vi "punto2.vi"() -> ()   [LabVIEW 2022 SP3]
uses:
  <vilib>/Instr/_visa.llb/VISA Configure Serial Port (Instr).vi
  <vilib>/addons/control/pid/pid.llb/PID (DBL).vi
  <vilib>/addons/control/pid/NI_PID_pid.lvlib
panel:
  in  "Potencia Manual":i16 min=0 max=100 step=1
  in  "Modo":bool=TRUE
  out "Input":cluster{i16}(graph)
  out "Velocidad":i32
  in  "PID gains":T1={"proportional gain (Kc)"=0.8, "integral time (Ti, min)"=0.053, "derivative time (Td, min)"=0.0} {"derivative time (Td, min)" format="%.3f"; "integral time (Ti, min)" format="%.3f"; "proportional gain (Kc)" format="%.3f"}
  in  "VISA resource name":refnum<visa-resource-name>
  in  "Stop Button":bool
  out "Output":cluster{i32, "Set Point":dbl}(graph)
  in  "Set Point":dbl
  # "INTEGRANTES"
  # "- SEBASTIÁN ALZATE SIERRA \n- GRACHI GONZALEZ PULGARIN \n- PABLO GARCÍA SUÁREZ"
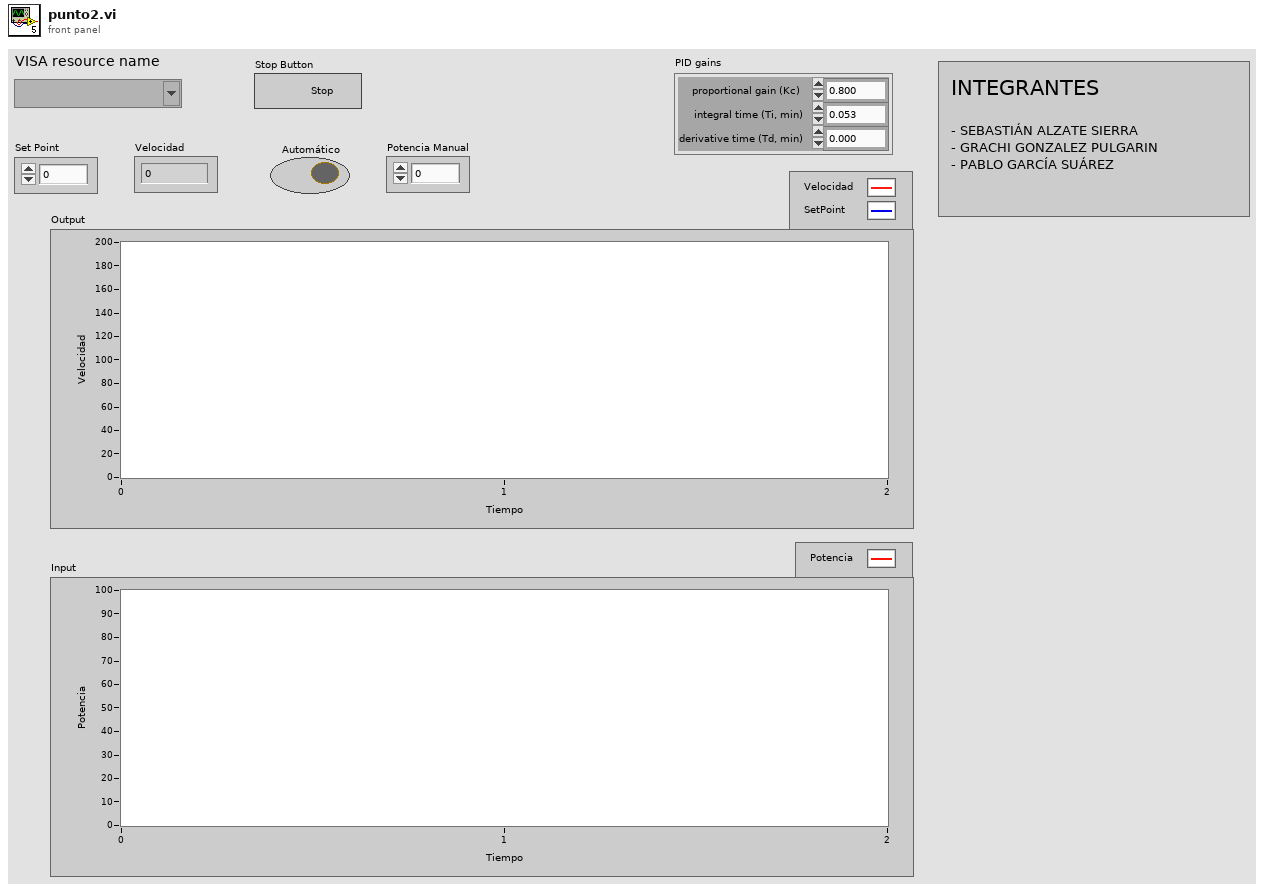
[diagram p1: front panel]
types:
  T1 = cluster{"proportional gain (Kc)":dbl, "integral time (Ti, min)":dbl, "derivative time (Td, min)":dbl}
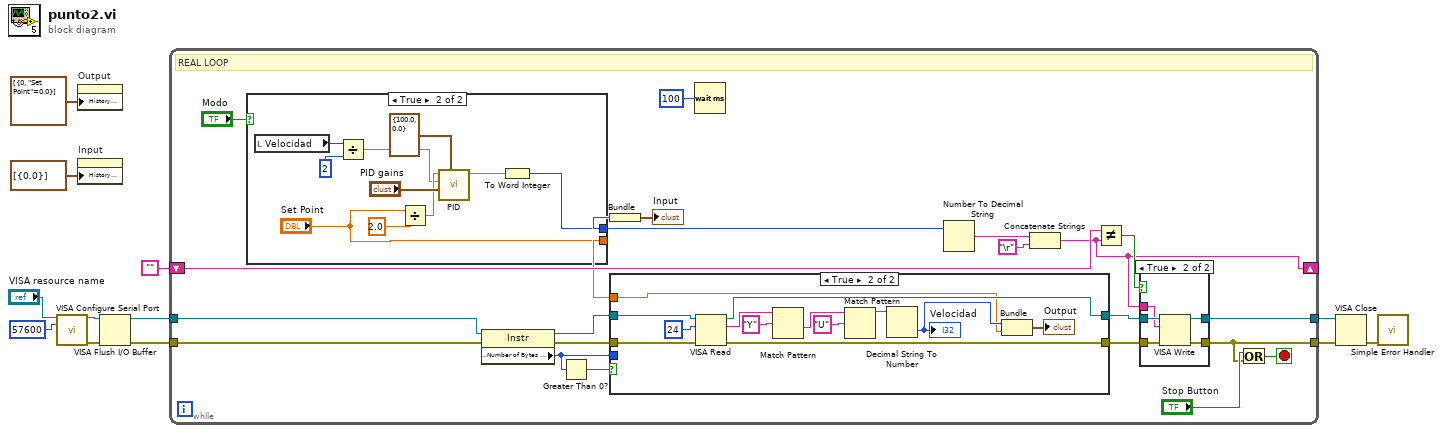
[diagram p0: block diagram]
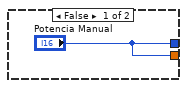
[diagram p2: hidden frame]
diagram:
  n1 = call-poly "VISA Configure Serial Port"("VISA resource name"="VISA resource name", "baud rate (9600)"=u32 57600) -> ("VISA resource name out"=w6:refnum<visa-resource-name>, "error out"=w5:errorcluster)  [unwired: 12 in]
  n2 = property on="Output" class="WFChart (strict)"("History Data"=cluster{i32, "Set Point":dbl}[] [{0, "Set Point"=0.0}]) -> ()  [unwired: 2 in, 2 out]
  n3 = property on="Input" class="WFChart (strict)"("History Data"=cluster{"output":dbl}[] [{"output"=0.0}]) -> ()  [unwired: 2 in, 2 out]
  n4 = VISA Flush I/O Buffer(VISA resource name=w6, error in (no error)=w5) -> (VISA resource name out=w4:refnum<visa-resource-name>, error out=w3:errorcluster)  [unwired: 1 in]
  n5 = while {
    tunnel: [w34] -> w12
    tunnel: [w27] -> w11
    shift-right: [w30] -> _
    shift-left: "" -> [w31]
    tunnel: w4 -> [w26]
    tunnel: w3 -> [w25]
    stop <- w33 stop-if-true
    # "REAL LOOP"
    n6 = case shown="True" "Modo" {
      tunnel: ["Potencia Manual" "Set Point"] -> w16
      tunnel: ["Potencia Manual" w42] -> w14
      frame False {
      }
      frame True {
        n7 = local read "Velocidad"() -> (w38:i32)
        n8 = Divide(x=w38, y=2) -> (x/y=w36:dbl)
        n9 = Divide(x="Set Point", y=2.0) -> (x/y=w40:dbl)
        n10 = call-poly <vilib>:"PID.vi"("output range"=cluster{"output high":dbl, "output low":dbl} {"output high"=100.0, "output low"=0.0}, "PID gains"="PID gains", "process variable"=w36, "setpoint"=w40) -> ("output"=w43:dbl)  [unwired: 6 in, 1 out]
        n11 = To Word Integer(number=w43) -> (16bit integer=w42:i16)
      }
    }
    n12 = property class="Instr"(reference=w26, error in=w25) -> (reference out=w24:refnum<visa-resource-name>, error out=w23:errorcluster, "Serial Settings:Number of Bytes at Serial Port"=w18:u32)
    n13 = Greater Than 0?(x=w18) -> (x > 0?=w20:bool)
    n14 = Bundle("Potencia Manual"=w14) -> (→"Input":cluster{"Potencia Manual":i16})  [unwired: 1 in]
    n15 = case shown="True" w20 {
      tunnel: w24 -> [w47 w60]
      tunnel: w23 -> [w46 w59]
      tunnel: [w47 w58] -> w22
      tunnel: [w46 w57] -> w21
      tunnel: w18 -> [_ _]
      tunnel: w16 -> [_ w48]
      frame False {
      }
      frame True {
        n16 = VISA Read(VISA resource name=w60, byte count=u32 24, error in (no error)=w59) -> (VISA resource name out=w58:refnum<visa-resource-name>, read buffer=w55:string, error out=w57:errorcluster)  [unwired: 1 out]
        n17 = Match Pattern(string=w55, regular expression="Y") -> (after substring=w51:string)  [unwired: 1 in, 3 out]
        n18 = Match Pattern(string=w51, regular expression="U") -> (before substring=w50:string)  [unwired: 1 in, 3 out]
        n19 = Decimal String To Number(string=w50) -> (number=w53:i32)  [unwired: 2 in, 1 out]
        "Velocidad" <- w53
        n20 = Bundle(w53, "Set Point"=w48) -> (→"Output":cluster{i32, "Set Point":dbl})  [unwired: 1 in]
      }
    }
    n21 = Wait (ms)(milliseconds to wait=u32 100) -> ()  [unwired: 1 out]
    n22 = Number To Decimal String(number=w14) -> (decimal integer string=w17:string)  [unwired: 1 in]
    n23 = Concatenate Strings(w17, "\r") -> (w30:string)
    n24 = Not Equal?(x=w31, y=w30) -> (x != y?=w32:bool)
    n25 = case shown="True" w32 {
      tunnel: w22 -> [w62 w67]
      tunnel: [w62 w66] -> w34
      tunnel: w21 -> [w61 w65]
      tunnel: [w61 w64] -> w27
      tunnel: w30 -> [_ w63]
      frame False {
      }
      frame True {
        n26 = VISA Write(VISA resource name=w67, write buffer=w63, error in (no error)=w65) -> (VISA resource name out=w66:refnum<visa-resource-name>, error out=w64:errorcluster)  [unwired: 1 out]
      }
    }
    n27 = Or(x="Stop Button", y=w27) -> (x .or. y?=w33:bool)
  }
  n28 = VISA Close(VISA resource name=w12, error in (no error)=w11) -> (error out=w9:errorcluster)
  n29 = call <vilib>:"Simple Error Handler.vi"("error in (no error)"=w9) -> ()  [unwired: 4 in, 5 out]
